vi "Set Min ROI Overlay.vi"(8 "error in (no error)":errorcluster, 10 "Min Gauge ROI":T2, 11 "Image in":T1) -> (0 "error out":errorcluster, 3 "Image out":T1)   [LabVIEW 2011, in "Meter Detection Custom Device.lvlib"]
uses:
  Meter Detection Custom Device.lvlib
  <vilib>/vision/Image Controls.llb/IMAQ Image.ctl
  Meter Detection Global Variable.vi
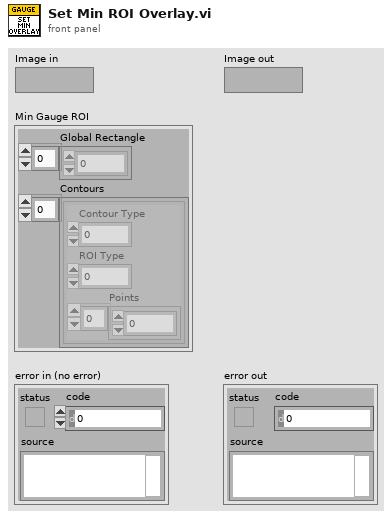
[diagram p1: front panel]
types:
  T1 = typedef "IMAQ Image.ctl" = refnum<image>
  T2 = cluster{"Global Rectangle":i32[], "Contours":cluster{"Contour Type":u32, "ROI Type":u32, "Points":i32[]}[]}
  T3 = cluster{"Desired Font (Application)":enum16{"User-specified Font", "Application Font", "System Font", "Dialog Font"}, "[User-specified Font]":cluster{"Font Name":string, "Size":i16, "Strikeout?":bool, "Italic?":bool, "Underline?":bool, "Outline?":bool, "Shadow?":bool, "Bold?":bool, "Rotation Angle":dbl}, "Horizontal Alignment":i16, "Vertical Alignment":i16}
  T4 = typedef "IMAQ Line" = cluster{"Start X":i32, "Start Y":i32, "End X":i32, "End Y":i32}
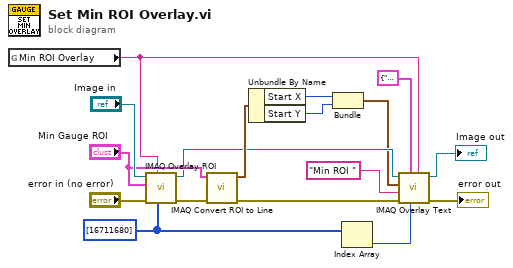
[diagram p0: block diagram]
diagram:
  w3 = u32[] [16711680] ("Colors (Green)")
  n1 = global read "Meter Detection Global Variable.vi" "Min ROI Overlay"() -> (w4:string)
  n2 = call "IMAQ Overlay ROI"("Colors (Green)"=w3, "Group"=w4, "error in (no error)"="error in (no error)", "ROI Descriptor"="Min Gauge ROI", "Image"="Image in") -> ("error out"=w12:errorcluster, "Image Out"=w7:T1)  [unwired: 5 in]
  n3 = call "IMAQ Convert ROI to Line"("error in (no error)"=w12, "ROI Descriptor"="Min Gauge ROI") -> ("error out"=w10:errorcluster, "Line"=w15:T4)  [unwired: 7 in]
  n4 = Unbundle By Name(w15) -> ("Start X"=w14:i32, "Start Y"=w13:i32)
  n5 = Bundle("Start X"=w14, "Start Y"=w13) -> (w5:cluster{"Start X":i32, "Start Y":i32})  [unwired: 1 in]
  n6 = Index Array(array=w3) -> (element=w2:u32)  [unwired: 1 in]
  n7 = call "IMAQ Overlay Text"("Group"=w4, "Text Color (black)"=w2, "Font, Size & Style"=T3 {"Desired Font (Application)"=enum."Application Font", "[User-specified Font]"={"Font Name"="", "Size"=12, "Strikeout?"=FALSE, "Italic?"=FALSE, "Underline?"=FALSE, "Outline?"=FALSE, "Shadow?"=FALSE, "Bold?"=FALSE, "Rotation Angle"=0.0}, "Horizontal Alignment"=1, "Vertical Alignment"=0}, "error in (no error)"=w10, "String"="Min ROI ", "Origin"=w5, "Image"=w7) -> ("error out"=→"error out":errorcluster, "Image Out"=→"Image out":T1)  [unwired: 3 in]
